vi "general.timestamp.vi"() -> (3 "timestamp":string)   [LabVIEW 2011]
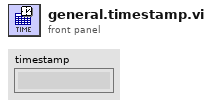
[diagram p1: front panel]
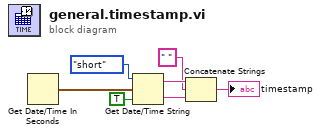
[diagram p0: block diagram]
diagram:
  n1 = Get Date/Time In Seconds() -> (seconds since 1Jan1904=w7:timestamp)
  n2 = Get Date/Time String(date format (0)=enum16{"short", "long", "abbreviated"}."short", seconds (now)=w7, want seconds? (F)=TRUE) -> (date string=w4:string, time string=w3:string)
  n3 = Concatenate Strings(w4, " " ("string"), w3) -> (→"timestamp":string)
